vi "get_setpoint.vi"(8 "error in (no error)":errorcluster, 10 "channel":dbl, 11 "Simulated_Instrument in":refnum<class "Simulated_Instrument.lvclass">) -> (0 "error out":errorcluster, 2 "setpoint":string, 3 "Simulated_Instrument out":refnum<class "Simulated_Instrument.lvclass">)   [LabVIEW 2018, in "Simulated_Instrument.lvclass"]
uses:
  Simulated_Instrument.lvclass
  instrument.lvclass
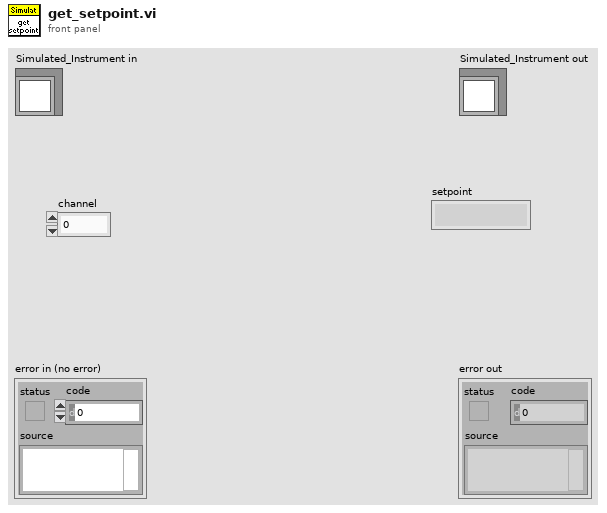
[diagram p1: front panel]
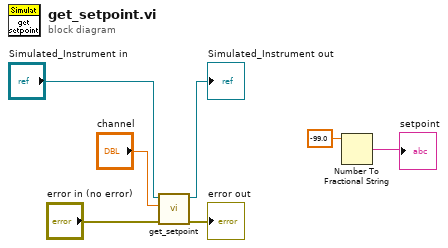
[diagram p0: block diagram]
diagram:
  n1 = call-parent "get_setpoint.vi"("error in (no error)"="error in (no error)", "channel"="channel", "instrument in"="Simulated_Instrument in") -> ("error out"=→"error out":errorcluster, "instrument out"=→"Simulated_Instrument out":refnum<class "Simulated_Instrument.lvclass">)  [unwired: 6 in, 1 out]
  n2 = Number To Fractional String(number=-99.0) -> (F-format string=→"setpoint":string)  [unwired: 3 in]
